vi "Script_Timing_Extract_Table_From_Text.vi"(7 "Script Text":string="script Pirenea2Excits1Acq4s\n   wait until scriptTrigger0 \n   wait 949940\n   generate AutLaserOn\n   wait 49000\n   generate AutLaserOnFilterOff\n   wait 1000\n   wait 600\n   generate AutLaserOnFilterOffTrapStart\n   wait 300\n   generate AutLaserOnFilterOffTrapStop\n   wait 2000\n   generate AutLaserOnFilterOn\n   wait 47100\n   generate AutLaserOff\n   wait 3950000\n   generate Excit\n   wait 1200\n   generate Excit\n   wait 1200\n   generate Acq\n   wait 1000000\n   generate FilterOff\n   wait 1000\n   generate FilterOffEmptyingStart\n   wait 1000000\n   generate FilterOffEmptyingStop\n   wait 2000\n   generate Zeros\nend script", 8 "error in (no error)":errorcluster, 10 "Script File":string="Pirenea2Excits1Acq4s.txt", 11 "Script Path":path=path "D:/PIRENEA/TECHNICAL/TIMING_SCRIPTS") -> (0 "error out":errorcluster, 2 "Script Text Cleaned":string, 3 "Table of Wfms":string[](array[string]))   [LabVIEW 2017]
uses:
  controls/TIMING_Table.ctl
  controls/TIMING_Mandatory_Items.ctl
  controls/TIMING_Optional_Items.ctl
  Global_Variables.vi
  <vilib>/regexp/Match Regular Expression.xnode
panel:
  in  "TIMING Table":T1={"Mandatory Items"={"Script Name"="", "HSDIO Delay"=60.0, "Shutter Delay before"=50.0, "Shutter Delay after"=50.0, "Filter Tau"=2.0, "Trapping Delay"=600.0, "Trapping Duration"=300.0, "Emtyping Duration"=1000.0}, "Optional Items"={"Eject"=0, "Acq"=0, "Excit"=0, "Gas"=0, "Laser"=0, "Lamp"=0}, "Times Table"=[["Excit1", "name", "Swift", "0.5", "1200", "70", "150", "550", "0", "0", "0"]]} {"Optional Items"."Laser" min=0 max=3; "Optional Items"."Gas" min=0 max=5; "Mandatory Items"."Shutter Delay after" min=10.0 max=200.0; "Mandatory Items"."HSDIO Delay" min=60.0 max=100.0; "Mandatory Items"."Shutter Delay before" min=10.0 max=200.0; "Mandatory Items"."Filter Tau" min=1.0 max=5.0; "Mandatory Items"."Trapping Delay" min=2.0 max=2000.0; "Mandatory Items"."Emtyping Duration" min=1.0 max=2000.0; "Mandatory Items"."Trapping Duration" min=2.0 max=2000.0}
  out "Table of Waits":string[](array[string])
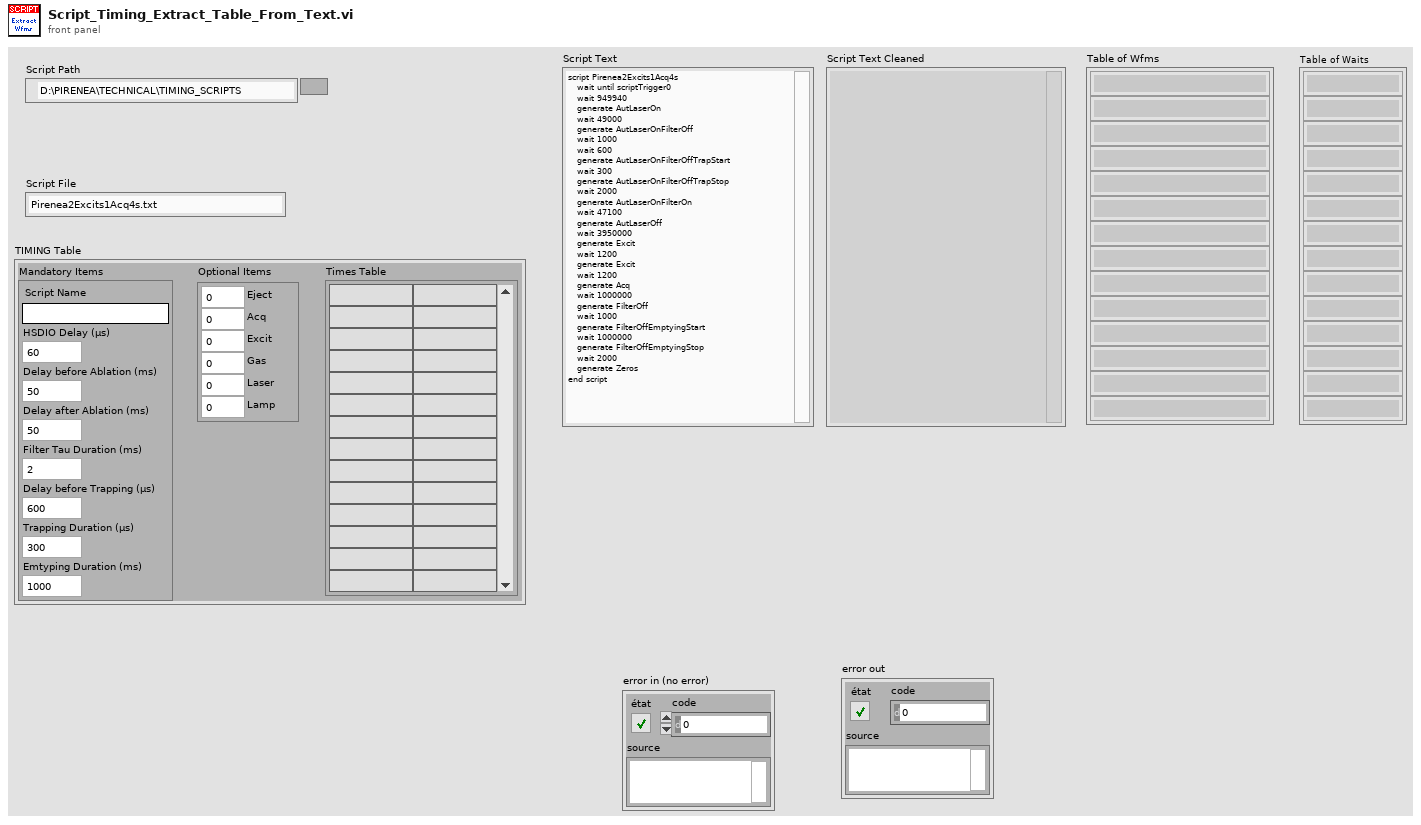
[diagram p1: front panel]
types:
  T1 = typedef "TIMING_Table.ctl" = cluster{"Mandatory Items":T2, "Optional Items":T3, "Times Table":string[][]}
  T2 = typedef "TIMING_Mandatory_Items.ctl" = cluster{"Script Name":string, "HSDIO Delay":dbl, "Shutter Delay before":dbl, "Shutter Delay after":dbl, "Filter Tau":dbl, "Trapping Delay":dbl, "Trapping Duration":dbl, "Emtyping Duration":dbl}
  T3 = typedef "TIMING_Optional_Items.ctl" = cluster{"Eject":u32, "Acq":i32, "Excit":u32, "Gas":i32, "Laser":i32, "Lamp":i32}
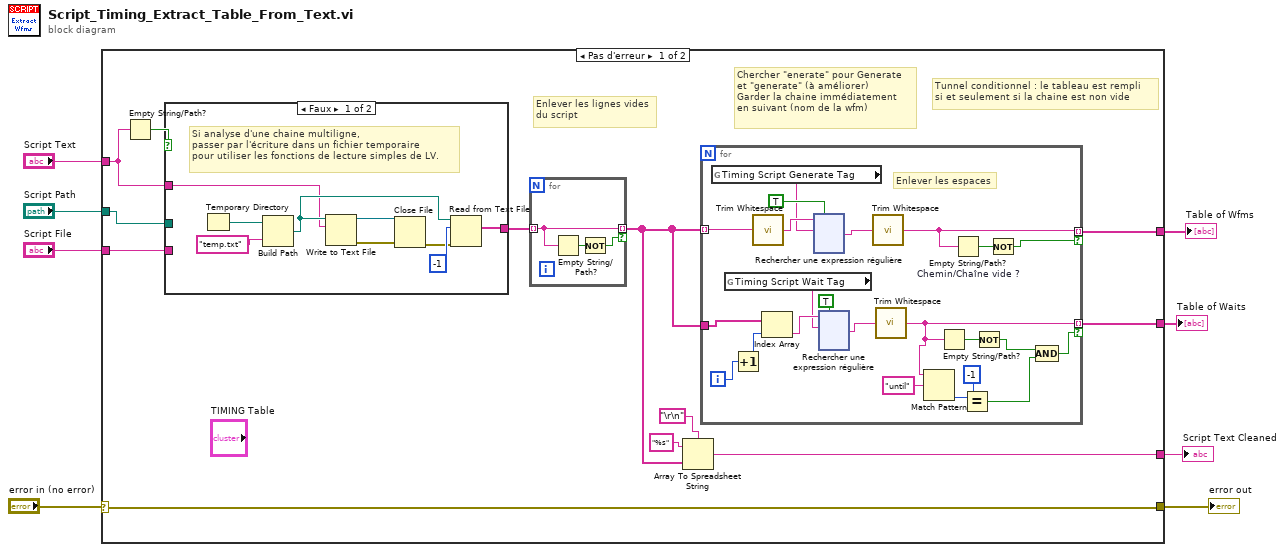
[diagram p0: block diagram]
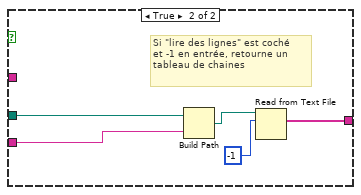
[diagram p2: hidden frame]
diagram:
  n1 = case shown="Pas d'erreur" "error in (no error)" {
    selector: "error in (no error)" -> [w11 w289]
    tunnel: [w19 _] -> w8
    tunnel: "Script Text" -> [w16 _]
    tunnel: [w14 _] -> w6
    tunnel: "Script Path" -> [w12 _]
    tunnel: "Script File" -> [w13 _]
    tunnel: [w11 w289] -> w3
    tunnel: [w9 _] -> w1
    frame No Error {
      # "Enlever les lignes vides\ndu script"
      # "Tunnel conditionnel : le tableau est rempli\nsi et seulement si la chaine est non vide"
      # "Chercher \"enerate\" pour Generate\net \"generate\" (à améliorer)\nGarder la chaine immédiatement\nen suivant (nom de la wfm)"
      n2 = Empty String/Path?(string/path=w16) -> (empty?=w15:bool)
      n3 = case shown="Faux" w15 {
        tunnel: w13 -> [_ w37]
        tunnel: w12 -> [_ w36]
        tunnel: [w24 w33] -> w17
        tunnel: w16 -> [w25 _]
        frame False {
          # "Si analyse d'une chaine multiligne,\npasser par l'écriture dans un fichier temporaire\npour utiliser les fonctions de lecture simples de LV."
          n4 = Temporary Directory() -> (w31:path)
          n5 = Build Path(base path=w31, name or relative path="temp.txt" ("nom ou chemin relatif")) -> (appended path=w28:path)
          n6 = Write to Text File(file (use dialog)=w28, text=w25) -> (refnum out=w29:refnum<file>, error out=w30:errorcluster)  [unwired: 2 in, 1 out]
          n7 = Close File(refnum=w29, error in=w30) -> (error out=w26:errorcluster)  [unwired: 1 out]
          n8 = Read from Text File(file (use dialog)=w28, count=-1 ("nombre"), error in=w26) -> (text=w24:string[])  [unwired: 1 in, 3 out]
        }
        frame True {
          # "Si \"lire des lignes\" est coché\net -1 en entrée, retourne un tableau de chaines"
          n9 = Build Path(base path=w36, name or relative path=w37) -> (appended path=w35:path)
          n10 = Read from Text File(file (use dialog)=w35, count=-1 ("nombre")) -> (text=w33:string[])  [unwired: 2 in, 3 out]
        }
      }
      n11 = for {
        tunnel: w17 -> [w22] mode=indexing
        tunnel: [w22] -> w10 mode=indexing if=w21
        n12 = Empty String/Path?(string/path=w22) -> (empty?=w23:bool)
        n13 = Not(x=w23) -> (.not. x?=w21:bool)
      }
      n14 = Array To Spreadsheet String(delimiter (Tab)="\r\n", array=w10, 3:"%s" ("chaîne de format")) -> (spreadsheet string=w19:string)
      n15 = for {
        tunnel: w10 -> [w60] mode=indexing
        tunnel: [w56] -> w14 mode=indexing if=w57
        tunnel: w10 -> [w52]
        tunnel: [w44] -> w9 mode=indexing if=w38
        i -> [w51]
        # "Enlever les espaces"
        n16 = global read "Global_Variables.vi" "Timing Script Generate Tag"() -> (w53:string)
        n17 = global read "Global_Variables.vi" "Timing Script Wait Tag"() -> (w48:string)
        n18 = Increment(x=w51) -> (x+1=w50:i32)
        n19 = call <vilib>:"Trim Whitespace.vi"("string"=w60) -> ("trimmed string"=w55:string)  [unwired: 1 in]
        n20 = Index Array(array=w52, index=w50) -> (element=w49:string)
        n21 = xnode "Rechercher une expression régulière"("chaîne en entrée"=w55, "expression régulière"=w53, "ignorer la casse ? (F)"=TRUE) -> ("après la correspondance"=w59:string)  [unwired: 3 in, 4 out]
        n22 = xnode "Rechercher une expression régulière"("chaîne en entrée"=w49, "expression régulière"=w48, "ignorer la casse ? (F)"=TRUE) -> ("après la correspondance"=w45:string)  [unwired: 3 in, 4 out]
        n23 = call <vilib>:"Trim Whitespace.vi"("string"=w59) -> ("trimmed string"=w56:string)  [unwired: 1 in]
        n24 = call <vilib>:"Trim Whitespace.vi"("string"=w45) -> ("trimmed string"=w44:string)  [unwired: 1 in]
        n25 = Match Pattern(string=w44, regular expression="until" ("expression régulière")) -> (offset past match=w42:i32)  [unwired: 1 in, 3 out]
        n26 = Empty String/Path? ("Chemin/Chaîne vide ?")(string/path=w44) -> (empty?=w46:bool)
        n27 = Empty String/Path? "Chemin/Chaîne vide ?"(string/path=w56) -> (empty?=w58:bool)
        n28 = Equal?(x=w42, y=-1) -> (x = y?=w40:bool)
        n29 = Not(x=w46) -> (.not. x?=w39:bool)
        n30 = Not(x=w58) -> (.not. x?=w57:bool)
        n31 = Compound Arithmetic op=AND ("Opérateur arithmétique")(w39, w40) -> (w38:bool)
      }
    }
    frame Error {
    }
  }
  "Script Text Cleaned" <- w8
  "Table of Wfms" <- w6
  "error out" <- w3
  "Table of Waits" <- w1
